vi "Load Menu RTM.vi"(8 "error in (no error)":errorcluster, 10 "MenuRTMPath":path, 11 "Menu in":refnum<class "Menu.lvclass">) -> (0 "error out":errorcluster, 3 "Menu out":refnum<class "Menu.lvclass">)   [LabVIEW 2021, in "Menu.lvlib" / "Menu.lvclass"]
uses:
  Menu.lvclass
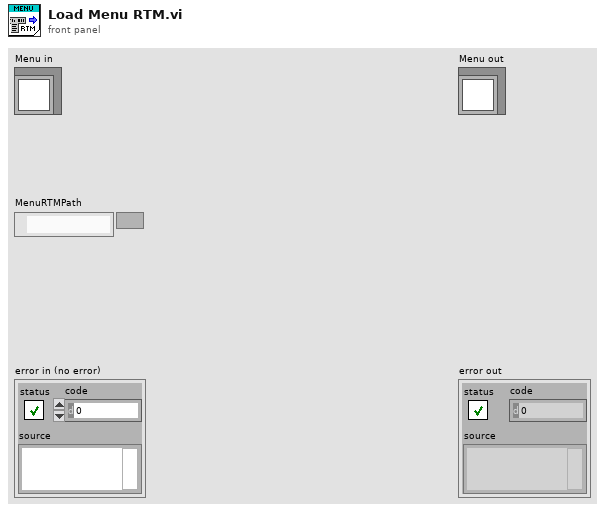
[diagram p1: front panel]
types:
  T1 = typedef "Menu.lvlib/Menu.lvclass/Data.ctl" = cluster{"MenuMap":map{string, T2}, "PictRef":refnum<vi>, "MenuSelectionEvent":refnum<user-event>, "TopMenuSpacing":i32, "MenuSpacing":i32, "CloseEvent":refnum<user-event>, "TR_ManageMenuRef":refnum<vi>, "MenuColors":T4, "RTMPath":path, "RTMVIReference":refnum<vi>, "RTMMenuReference":refnum<k9>, "CtlRef":refnum<vi>, "User-Specified Font":refnum<class "Font.lvclass">, "Desired Font":enum16{"User-specified Font", "Application Font", "System Font", "Dialog Font"}, "SubMenuIcon":T5, "SubMenuIconClosed":refnum<class "Picture2D.lvclass">, "SubMenuIconOpened":refnum<class "Picture2D.lvclass">}
  T2 = typedef "Menu.lvlib/Menu.lvclass/MenuItems.ctl" = cluster{"Item Name":string, "Short Cut":T3, "Checked":bool, "Enable":bool, "After item":string, "Item Tags":string[], "Item Names":string[], "Picture":refnum<class "Image.lvclass">, "Hilite Picture":refnum<class "Image.lvclass">, "Displayed":bool}
  T3 = typedef "LVMenuShortCut.ctl" = cluster{"Include Shift Key?":bool, "Include Ctrl Key?":bool, "Shortcut Key":string}
  T4 = typedef "Menu.lvlib/Menu.lvclass/MenuColors.ctl" = cluster{"Text":refnum<class "Color.lvclass">, "HiliteText":refnum<class "Color.lvclass">, "Background":refnum<class "Color.lvclass">, "BorderColor":refnum<class "Color.lvclass">, "Hilite":refnum<class "Color.lvclass">}
  T5 = typedef "Menu.lvlib/Menu.lvclass/SubMenuIcon.ctl" = enum16{"LabVIEW", "Windows", "Custom"}
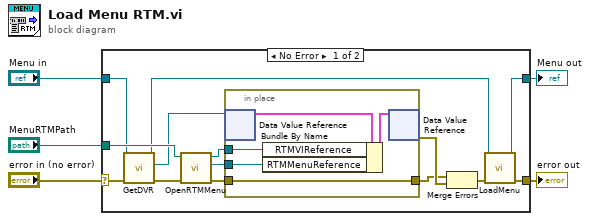
[diagram p0: block diagram]
diagram:
  n1 = case shown="No Error" "error in (no error)" {
    selector: "error in (no error)" -> [w18 w26]
    tunnel: [w12 w26] -> w4
    tunnel: [w6 w25] -> w2
    tunnel: "Menu in" -> [w8 w25]
    tunnel: "MenuRTMPath" -> [w19 _]
    frame No Error {
      n2 = call "GetDVR.vi"("error in (no error)"=w18, "Menu in"=w8) -> ("error out"=w17:errorcluster, "DVR"=w14:refnum<data-value>, "Menu out"=w7:refnum<class "Menu.lvclass">)  [unwired: 7 in]
      n3 = call "OpenRTMMenu.vi"("error in"=w17, "RTMFilePath"=w19) -> ("error out"=w9:errorcluster, "RTMMenuReference"=w10:refnum<k9>, "RTMVIReference"=w11:refnum<vi>)  [unwired: 7 in]
      n4 = in-place {
        in-place-border: w9 -> [w20]
        in-place-border: [w20] -> w15
        in-place-border: w11 -> [w22]
        in-place-border: w10 -> [w21]
        n5 = in-place-dvr #1(w14) -> (w23:T1)  [unwired: 1 out]
        n6 = Bundle By Name(cluster=w23, "RTMVIReference"=w22, "RTMMenuReference"=w21) -> (w24:T1)
        n7 = in-place-dvr #1(w24) -> (w16:errorcluster)  [unwired: 1 out]
      }
      n8 = Merge Errors(w15, w16) -> (w13:errorcluster)
      n9 = call "LoadMenu.vi"("error in (no error)"=w13, "Menu in"=w7) -> ("error out"=w12:errorcluster, "Menu out"=w6:refnum<class "Menu.lvclass">)  [unwired: 8 in]
    }
    frame Error {
    }
  }
  "error out" <- w4
  "Menu out" <- w2
